vi "subvi.vi"(8 "cluster in":T1, 9 "Boolean":bool=TRUE, 10 "Numeric":i32, 11 "String":string) -> ()   [LabVIEW 2015]
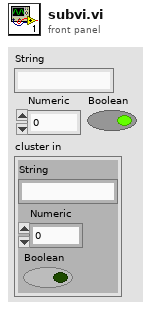
[diagram p1: front panel]
types:
  T1 = cluster{"String":string, "Numeric":i32, "Boolean":bool}
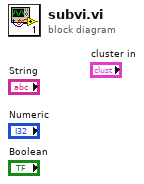
[diagram p0: block diagram]
diagram:
